vi "Recieve Register for Timer Events.vi"(8 "error in (no error)":errorcluster, 9 "Name":string, 10 "Timer period, -1  deafault":dbl=-1.0, 11 "Measurement Timer in":refnum<class "Measurement Timer.lvclass">) -> (0 "error out":errorcluster, 3 "Measurement Timer out":refnum<class "Measurement Timer.lvclass">)   [LabVIEW 2015, in "Measurement Timer.lvclass"]
uses:
  Measurement Timer.lvclass
  Measurement Timer.lvclass/Measurement Timer.ctl
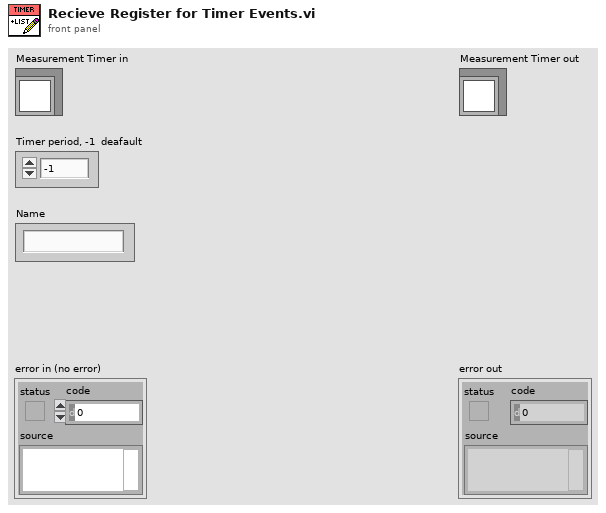
[diagram p1: front panel]
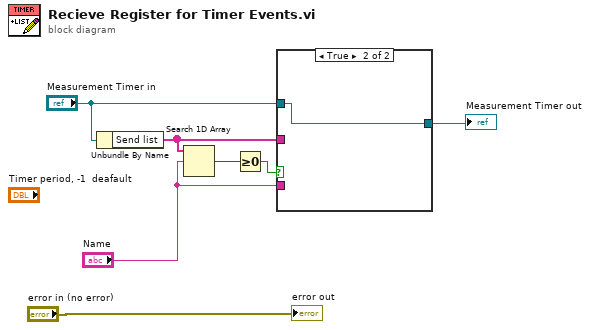
[diagram p0: block diagram]
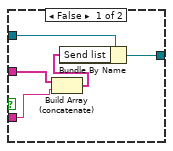
[diagram p2: hidden frame]
diagram:
  n1 = Unbundle By Name("Measurement Timer in") -> ("Send list"=w7:string[])
  n2 = Search 1D Array(1D array=w7, element="Name") -> (index of element=w6:i32)  [unwired: 1 in]
  n3 = Greater Or Equal To 0?(x=w6) -> (x >= 0?=w4:bool)
  n4 = case shown="True" w4 {
    tunnel: w7 -> [w12 _]
    tunnel: "Name" -> [w11 _]
    tunnel: "Measurement Timer in" -> [w10 w13]
    tunnel: [w8 w13] -> w2
    frame False {
      n5 = Build Array (concatenate)(w12, w11) -> (w9:string[])
      n6 = Bundle By Name(cluster=w10, "Send list"=w9) -> (w8:refnum<class "Measurement Timer.lvclass">)
    }
    frame True {
    }
  }
  "Measurement Timer out" <- w2
  "error out" <- "error in (no error)"
